vi "From Variant.vi"(8 "Error In":errorcluster, 10 "Variant":variant, 11 "TD Error Cluster In":refnum<class "Error Cluster.lvclass">) -> (0 "Error Out":errorcluster, 3 "TD Error Cluster Out":refnum<class "Error Cluster.lvclass">)   [LabVIEW 2017, in "Tree API.lvlib" / "Error Cluster.lvclass"]
doc: "Dynamic dispatch interface for conversion of variant LV data to Tree Data classes."
uses:
  Error Cluster.lvclass
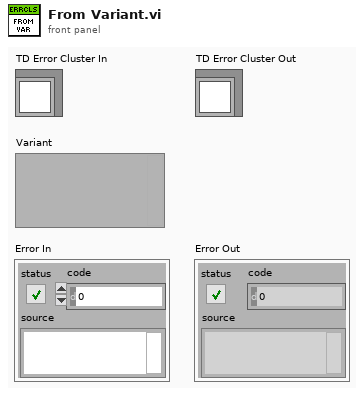
[diagram p1: front panel]
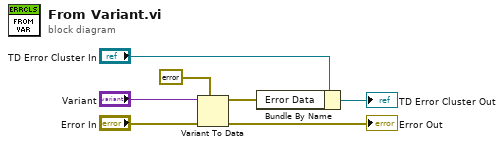
[diagram p0: block diagram]
diagram:
  n1 = Variant To Data(error in="Error In", type=errorcluster {"status"=FALSE, "code"=0, "source"=""} ("Error In"), Variant="Variant") -> (data=w3:errorcluster, error out=→"Error Out":errorcluster)
  n2 = Bundle By Name(cluster="TD Error Cluster In", "Error Data"=w3) -> (→"TD Error Cluster Out":refnum<class "Error Cluster.lvclass">)
